vi "Import EPT Pattern from File.vi"(8 "error in (no error)":errorcluster, 9 "Protocol in":string, 10 "Path":path, 11 "Class Lookup":variant) -> (0 "error out":errorcluster, 2 "EPT Pattern":T1, 3 "Class Lookup out":variant)   [LabVIEW 2017, in "Engine Simulation Toolkit System Explorer.lvlib"]
uses:
  Engine Simulation Toolkit System Explorer.lvlib
  File Formats.lvlibp/Parent/FileFormat.lvclass
  File Formats.lvlibp/Parent/EST Pattern.ctl
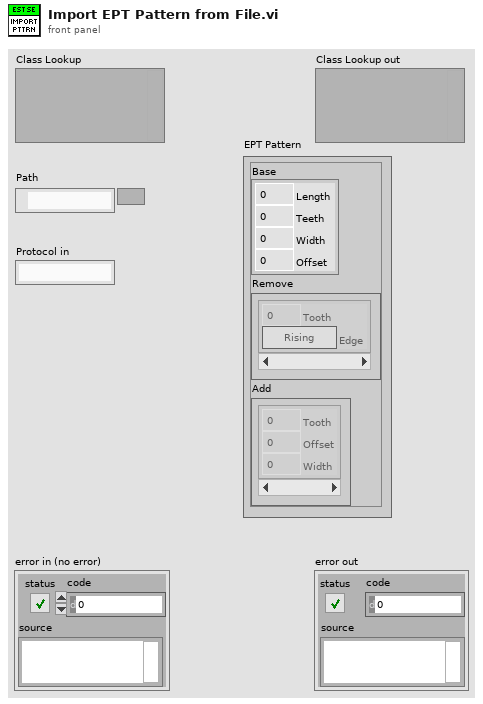
[diagram p1: front panel]
types:
  T1 = typedef "File Formats.lvlibp/FileFormat.lvclass/EST Pattern.ctl" = cluster{"Base":cluster{"Length":dbl, "Teeth":u16, "Width":dbl, "Offset":dbl}, "Remove":cluster{"Tooth":u16, "Edge":bool}[], "Add":cluster{"Tooth":u16, "Offset":dbl, "Width":dbl}[]}
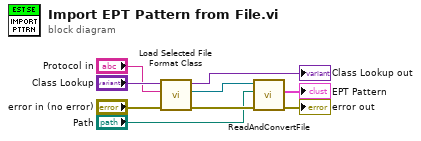
[diagram p0: block diagram]
diagram:
  n1 = call "Load Selected File Format Class.vi"("error in (no error)"="error in (no error)", "Protocol in"="Protocol in", "Class Lookup"="Class Lookup") -> ("error out"=w8:errorcluster, "FileFormat.lvclass"=w3:refnum<class "FileFormat.lvclass">, "Class Lookup"=→"Class Lookup out":variant)  [unwired: 6 in]
  n2 = call-dynamic "ReadAndConvertFile.vi"("error in (no error)"=w8, "Path"="Path", "FileFormat in"=w3) -> ("error out"=→"error out":errorcluster, "EPT Pattern"=→"EPT Pattern":T1)  [unwired: 6 in, 1 out]
